vi "generator_point_by_point(SubVI).vi"(6 "Amp":dbl, 7 "Numeric":dbl, 8 "offset":dbl, 9 "phase":dbl, 10 "freq":dbl, 11 "Sygnal":T1(ring)) -> (3 "Gaussian white noise":dbl)   [LabVIEW 2025]
uses:
  <vilib>/ptbypt/NI_PtbyPt.lvlib
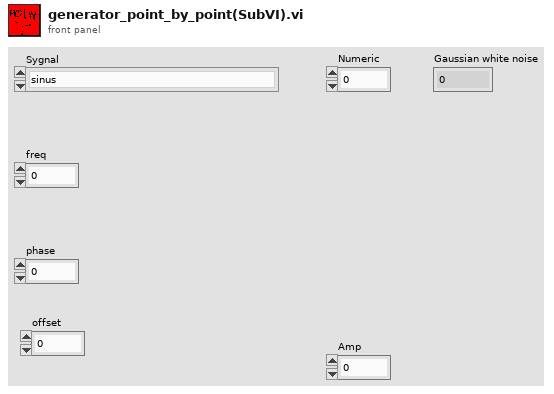
[diagram p1: front panel]
types:
  T1 = enum16{"sinus", "prostokat", "pila", "trojkat", "rozklad losowy", "rozklad normalny"}
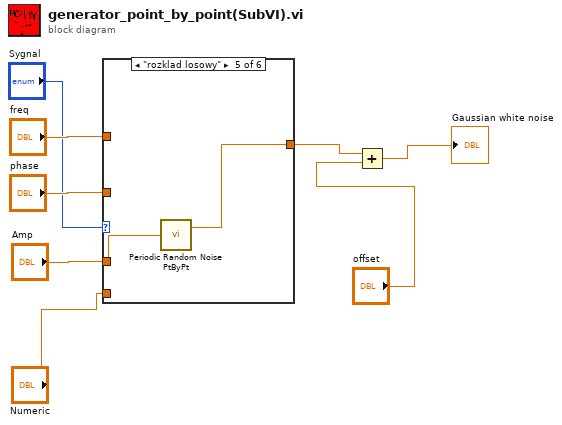
[diagram p0: block diagram]
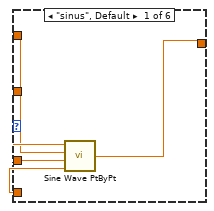
[diagram p2: hidden frame]
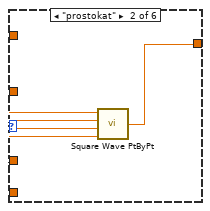
[diagram p3: hidden frame]
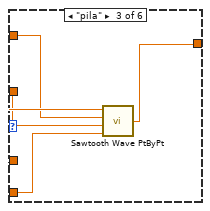
[diagram p4: hidden frame]
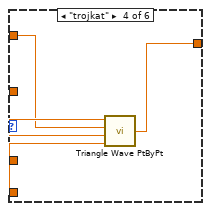
[diagram p5: hidden frame]
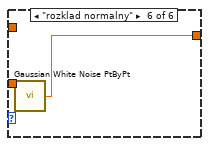
[diagram p6: hidden frame]
diagram:
  n1 = case shown="\"rozklad losowy\"" "Sygnal" {
    tunnel: [w13 w18 w23 w28 w30 w31] -> w3
    tunnel: "Amp" -> [w12 w14 w22 w27 w29 _]
    tunnel: "freq" -> [w11 w17 w21 w26 _ _]
    tunnel: "phase" -> [w10 w16 w20 w24 _ _]
    tunnel: "Numeric" -> [w9 w15 w19 w25 _ _]
    frame "sinus", Default {
      n2 = call <vilib>:"Sine Wave PtByPt.vi"("time"=w9, "phase"=w10, "frequency"=w11, "amplitude"=w12) -> ("sine wave"=w13:dbl)
    }
    frame "prostokat" {
      n3 = call <vilib>:"Square Wave PtByPt.vi"("amplitude"=w14, "frequency"=w17, "phase"=w16, "time"=w15) -> ("square wave"=w18:dbl)  [unwired: 1 in]
    }
    frame "pila" {
      n4 = call <vilib>:"Sawtooth Wave PtByPt.vi"("time"=w19, "phase"=w20, "frequency"=w21, "amplitude"=w22) -> ("sawtooth wave"=w23:dbl)
    }
    frame "trojkat" {
      n5 = call <vilib>:"Triangle Wave PtByPt.vi"("time"=w25, "phase"=w24, "frequency"=w26, "amplitude"=w27) -> ("triangle wave"=w28:dbl)
    }
    frame "rozklad losowy" {
      n6 = call <vilib>:"Periodic Random Noise PtByPt.vi"("spectral amplitude"=w29) -> ("periodic random noise"=w30:dbl)  [unwired: 3 in, 1 out]
    }
    frame "rozklad normalny" {
      n7 = call <vilib>:"Gaussian White Noise PtByPt.vi"() -> ("Gaussian white noise"=w31:dbl)  [unwired: 3 in]
    }
  }
  n8 = Add(x=w3, y="offset") -> (x+y=→"Gaussian white noise":dbl)
